vi "set_temperature.vi"(1 "Temperature (C)":dbl) -> ()   [LabVIEW 2011]
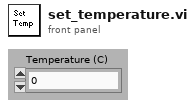
[diagram p1: front panel]
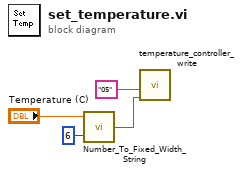
[diagram p0: block diagram]
diagram:
  n1 = call "Number_To_Fixed_Width_String.vi"("Width"=6, "Number"="Temperature (C)") -> ("String"=w1:string)
  n2 = call "temperature_controller_write.vi"("Value"=w1, "Command"="05") -> ()  [unwired: 2 in, 1 out]
